vi "Set Progress Value.vi"(7 "maximum (100)":u64=100, 8 "error in (no error)":errorcluster, 10 "current (0)":u64, 11 "Window Handle":refnum<k24>) -> (0 "error out":errorcluster, 3 "dup Window Handle":refnum<k24>)   [LabVIEW 2011, in "TaskbarProgressAPI.lvlib"]
doc: "Sets the current Progress bar value of the Progress bar embedded in the Taskbar button of the Window referenced by the Window Handle. The maximum corresponds to a fully filled progress bar. \n\nPlease see the 'LabVIEW Taskbar Progress Bar API Example.vi' in the NI Example finder for details on how to use this VI."
uses:
  TaskbarProgressAPI.lvlib
  C:/Users/nlvanzwk/Dropbox/LabVIEW/LabVIEW Tools Network/LabVIEW Taskbar Progress Bar API/LabVIEW Taskbar Progress Bar API/Windows7Taskbar.dll
  Windows7Taskbar.dll
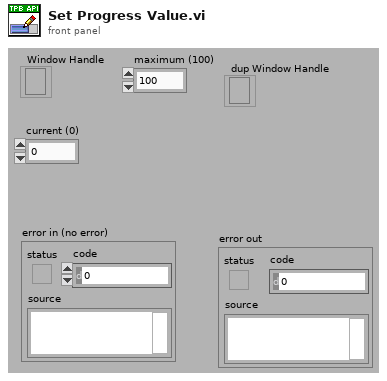
[diagram p1: front panel]
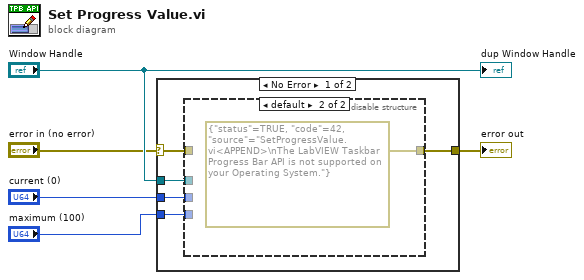
[diagram p0: block diagram]
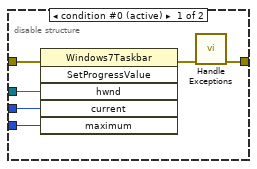
[diagram p2: hidden frame]
diagram:
  n1 = case shown="No Error" "error in (no error)" {
    selector: "error in (no error)" -> [w8 w18]
    tunnel: [w10 w18] -> w5
    tunnel: "Window Handle" -> [w9 _]
    tunnel: "current (0)" -> [w7 _]
    tunnel: "maximum (100)" -> [w6 _]
    frame No Error {
      n2 = disable-structure shown="default" {
        disable-tunnel: [w11 errorcluster {"status"=TRUE, "code"=42, "source"="SetProgressValue.vi<APPEND>\nThe LabVIEW Taskbar Progress Bar API is not supported on your Operating System."} ("error out")] -> w10
        disable-tunnel: w9 -> [w16 _]
        disable-tunnel: w8 -> [w15 _]
        disable-tunnel: w7 -> [w14 _]
        disable-tunnel: w6 -> [w13 _]
        frame condition #0 (active) {
          n3 = invoke class="Windows7Taskbar" method="SetProgressValue"(error in=w15, "hwnd"=w16, "current"=w14, "maximum"=w13) -> (error out=w12:errorcluster)  [unwired: 2 in, 5 out]
          n4 = call "Handle Exceptions.vi"("error in (no error)"=w12) -> ("error out"=w11:errorcluster)  [unwired: 10 in]
        }
        frame condition #1 {
        }
      }
    }
    frame Error {
    }
  }
  "error out" <- w5
  "dup Window Handle" <- "Window Handle"
